vi "duplicateNode.vi"(8 "error in (no error)":errorcluster, 10 "superNode*":refnum<data-value>, 11 "xceNode in":refnum<class "xceNode.lvclass">) -> (0 "error out":errorcluster, 2 "duplicateNode*":refnum<data-value>, 3 "xceNode out":refnum<class "xceNode.lvclass">)   [LabVIEW 2013, in "xceNode.lvclass"]
doc: "Duplicates a node, and adds it to the appropriate superNode."
uses:
  xceNode.lvclass
  xceTreeObj/xceTreeObj.lvclass
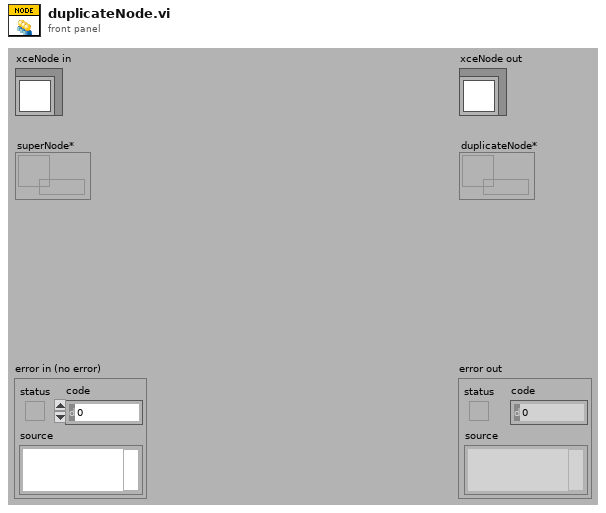
[diagram p1: front panel]
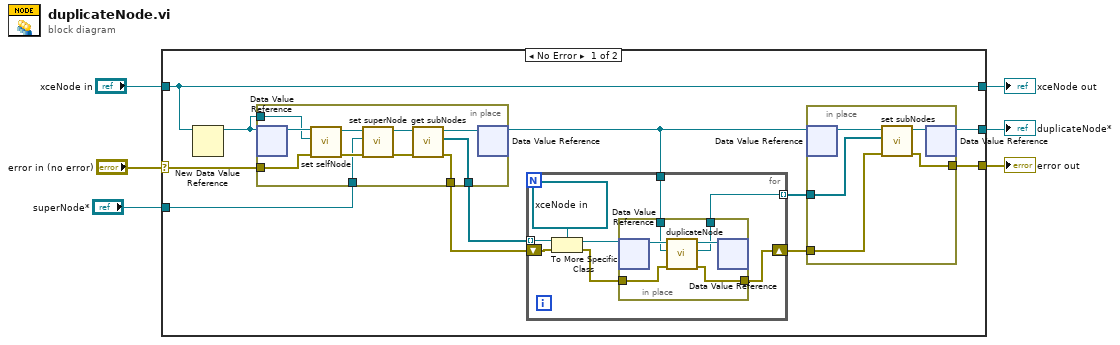
[diagram p0: block diagram]
diagram:
  n1 = case shown="No Error" "error in (no error)" {
    selector: "error in (no error)" -> [w9 w49]
    tunnel: [w8 w49] -> w5
    tunnel: [w17 w48] -> w3
    tunnel: "xceNode in" -> [w17 w48]
    tunnel: "superNode*" -> [w16 _]
    tunnel: [w10 _] -> w2
    frame No Error {
      n2 = New Data Value Reference(data value=w17) -> (data value reference=w7:refnum<data-value>)  [unwired: 1 in, 1 out]
      n3 = in-place {
        in-place-border: w7 -> [w46]
        in-place-border: w16 -> [w40]
        in-place-border: [w39] -> w15
        in-place-border: [w38] -> w14
        in-place-border: w9 -> [w37]
        n4 = in-place-dvr #1(w7) -> (w47:refnum<class "xceNode.lvclass">)  [unwired: 1 out]
        n5 = call "set selfNode.vi"("error in (no error)"=w37, "selfNode*"=w46, "xceNode in"=w47) -> ("error out"=w45:errorcluster, "xceNode out"=w44:refnum<class "xceNode.lvclass">)  [unwired: 7 in]
        n6 = call "set superNode.vi"("error in (no error)"=w45, "superNode*"=w40, "xceNode in"=w44) -> ("error out"=w41:errorcluster, "xceNode out"=w43:refnum<class "xceNode.lvclass">)  [unwired: 7 in]
        n7 = call "get subNodes.vi"("error in (no error)"=w41, "xceNode in"=w43) -> ("error out"=w38:errorcluster, "subNodes[]*"=w39:refnum<data-value>[], "xceNode out"=w42:refnum<class "xceNode.lvclass">)  [unwired: 7 in]
        n8 = in-place-dvr #1(w42) -> (w13:refnum<data-value>)  [unwired: 1 out]
      }
      n9 = for {
        tunnel: w15 -> [w30] mode=indexing
        tunnel: w13 -> [w27]
        shift-right: [w24] -> w12
        shift-left: w14 -> [w25]
        tunnel: [w23] -> w11 mode=indexing
        n10 = To More Specific Class(target class=refnum<data-value> refnum ("data value reference"), reference=w30, error in=w25) -> (specific class reference=w28:refnum<data-value>, error out=w26:errorcluster)
        n11 = in-place {
          in-place-border: w27 -> [w35]
          in-place-border: w26 -> [w34]
          in-place-border: [w33] -> w24
          in-place-border: [w31] -> w23
          n12 = in-place-dvr #2(w28) -> (w36:refnum<class "xceNode.lvclass">)  [unwired: 1 out]
          n13 = call "duplicateNode.vi"("error in (no error)"=w34, "superNode*"=w35, "xceNode in"=w36) -> ("error out"=w33:errorcluster, "duplicateNode*"=w31:refnum<data-value>, "xceNode out"=w32:refnum<class "xceNode.lvclass">)  [unwired: 6 in]
          n14 = in-place-dvr #2(w32) -> ()  [unwired: 2 out]
        }
      }
      n15 = in-place {
        in-place-border: w12 -> [w22]
        in-place-border: w11 -> [w20]
        in-place-border: [w18] -> w8
        n16 = in-place-dvr #3(w13) -> (w21:refnum<class "xceNode.lvclass">)  [unwired: 1 out]
        n17 = call "set subNodes.vi"("error in (no error)"=w22, "subNodes[]*"=w20, "xceNode in"=w21) -> ("error out"=w18:errorcluster, "xceNode out"=w19:refnum<class "xceNode.lvclass">)  [unwired: 7 in]
        n18 = in-place-dvr #3(w19) -> (w10:refnum<data-value>)  [unwired: 1 out]
      }
    }
    frame Error {
    }
  }
  "error out" <- w5
  "xceNode out" <- w3
  "duplicateNode*" <- w2
